vi "Shooter Control and protect.vi"(5 "Shoot":bool, 7 "Reset":bool, 8 "Auto Reset Delay (ms)":dbl, 9 "Target RPM":dbl, 10 "%VBus":dbl, 11 "Talon Status":T1) -> (1 "DISABLED":bool, 2 "Output":dbl, 3 "Control Mode":T2)   [LabVIEW 2016]
doc: "When the shoot terminal recives true the shooter shifts to speed mode and goes to the target speed. When the shoot terminal goes false the shooter stays on for Delay miliseconds. This prevents balls from entering the shooter while it's speed is too low.\n\nWhen the shoot terminal is false the shooter is in manual percent VBus mode.\n\nIf the shooter has stalled it will be disabled. When disabled the shooter will not move and can be re-enabled by sending true to the reset terminal.\n\nThe shooter can also be enabled by using the auto reset. When the Auto reset terminal is set to zero it will not auto reset. When the reset terminal is positive it will wait for The specified delay then set the reset terminal to true."
uses:
  <vilib>/Rock Robotics/WPI/ThirdParty/CanMotor/TalonSRX/WPI_CANTalonSRX_APIControlMode.ctl
  <vilib>/Rock Robotics/WPI/ThirdParty/CanMotor/TalonSRX/WPI_CANTalonSRX_GlobalStatus.ctl
  <vilib>/Rock Robotics/Network Tables/NT Read Boolean.vi
  Delay Polymorphic/Delay Boolean.vi
panel:
  in  "Delay (ms)":i32
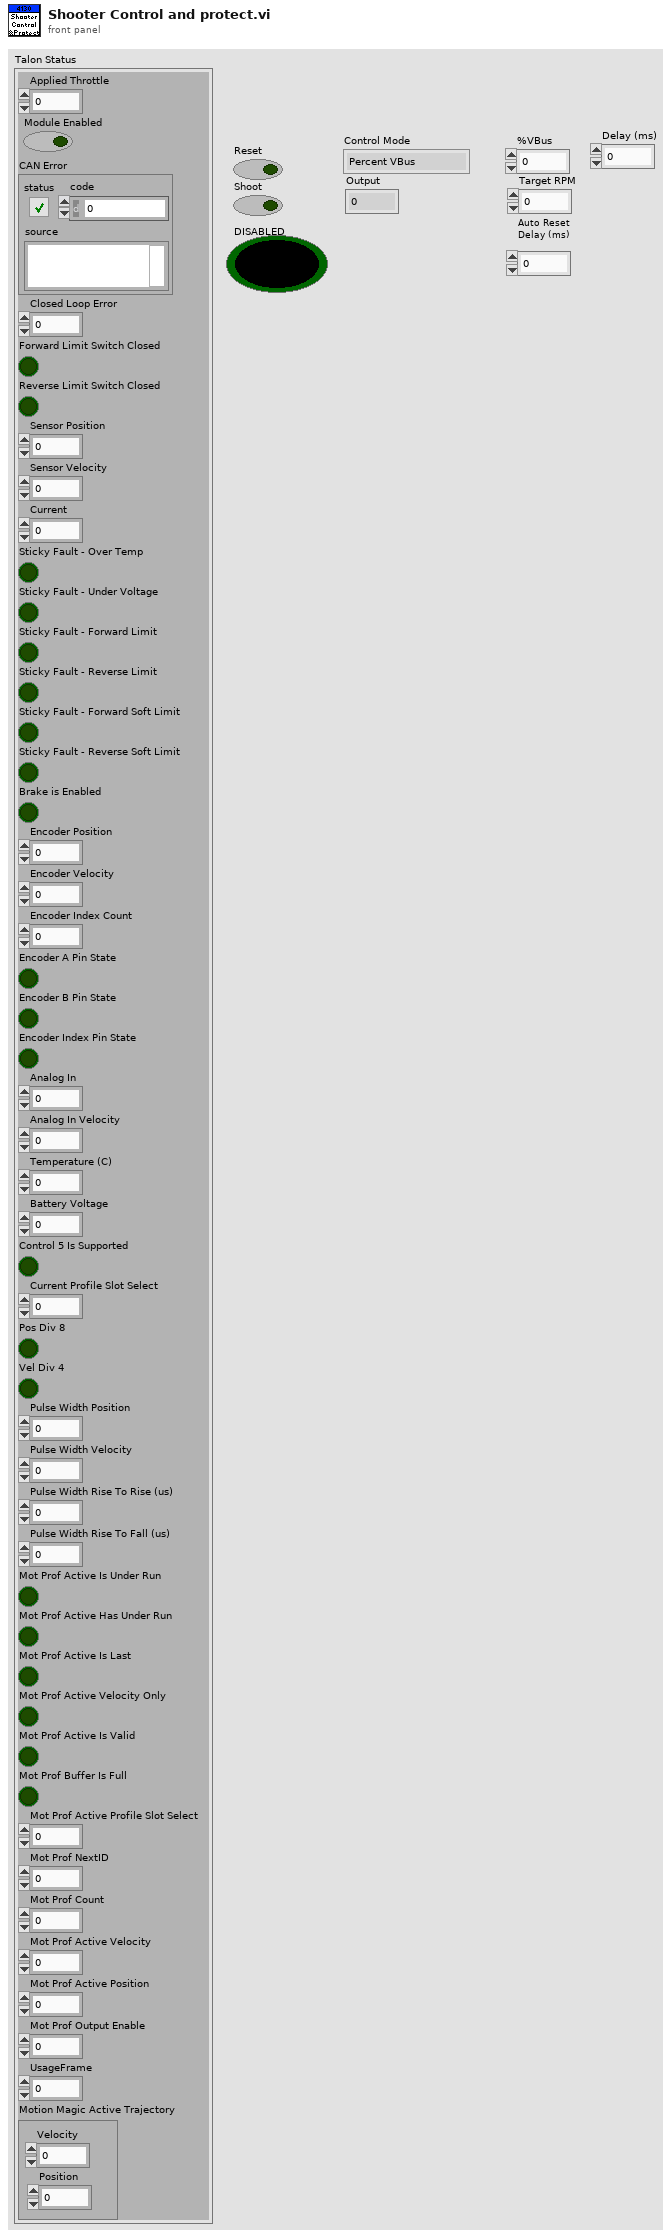
[diagram p1: front panel]
types:
  T1 = typedef "WPI_CANTalonSRX_GlobalStatus.ctl" = cluster{"Applied Throttle":dbl, "Module Enabled":bool, "CAN Error":errorcluster, "Closed Loop Error":dbl, "Forward Limit Switch Closed":bool, "Reverse Limit Switch Closed":bool, "Sensor Position":dbl, "Sensor Velocity":dbl, "Current":dbl, "Sticky Fault - Over Temp":bool, "Sticky Fault - Under Voltage":bool, "Sticky Fault - Forward Limit":bool, "Sticky Fault - Reverse Limit":bool, "Sticky Fault - Forward Soft Limit":bool, "Sticky Fault - Reverse Soft Limit":bool, "Brake is Enabled":bool, "Encoder Position":dbl, "Encoder Velocity":dbl, "Encoder Index Count":dbl, "Encoder A Pin State":bool, "Encoder B Pin State":bool, "Encoder Index Pin State":bool, "Analog In":dbl, "Analog In Velocity":dbl, "Temperature (C)":dbl, "Battery Voltage":dbl, "Control 5 Is Supported":bool, "Current Profile Slot Select":dbl, "Pos Div 8":bool, "Vel Div 4":bool, "Pulse Width Position":i32, "Pulse Width Velocity":i32, "Pulse Width Rise To Rise (us)":i32, "Pulse Width Rise To Fall (us)":i32, "Mot Prof Active Is Under Run":bool, "Mot Prof Active Has Under Run":bool, "Mot Prof Active Is Last":bool, "Mot Prof Active Velocity Only":bool, "Mot Prof Active Is Valid":bool, "Mot Prof Buffer Is Full":bool, "Mot Prof Active Profile Slot Select":i32, "Mot Prof NextID":i32, "Mot Prof Count":i32, "Mot Prof Active Velocity":dbl, "Mot Prof Active Position":dbl, "Mot Prof Output Enable":i32, "UsageFrame":u32, "Motion Magic Active Trajectory":cluster{"Velocity":dbl, "Position":dbl}}
  T2 = typedef "WPI_CANTalonSRX_APIControlMode.ctl" = enum8{"Percent VBus", "Speed", "Position", "Slave", "Unchanged / Invalid", "Voltage Compensation", "Current", "Motion Profile", "Motion Magic"}
  T3 = enum16{"Rising", "Falling", "Neither", "Instant"}
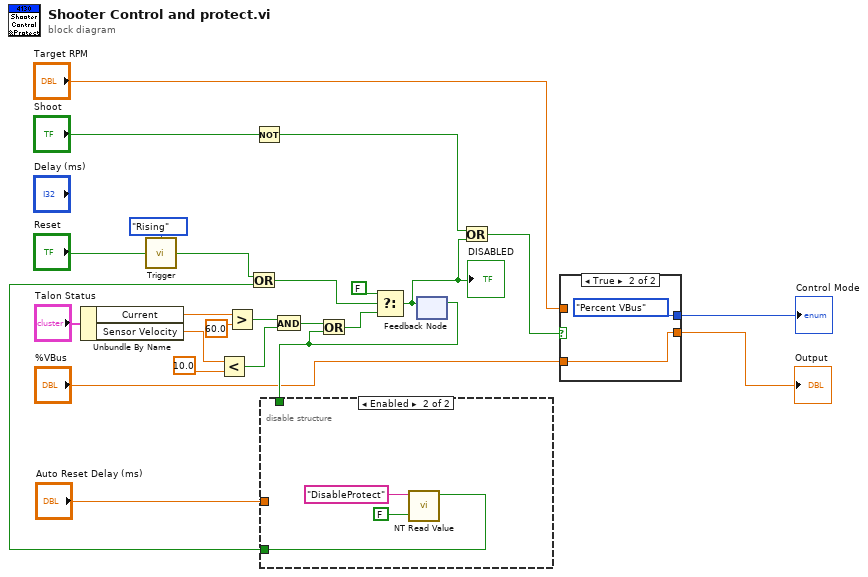
[diagram p0: block diagram]
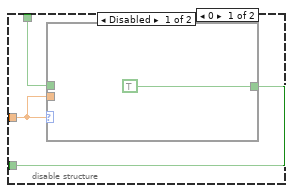
[diagram p2: hidden frame]
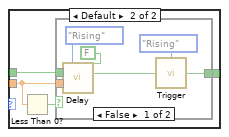
[diagram p3: hidden frame]
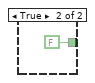
[diagram p4: hidden frame]
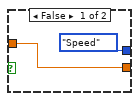
[diagram p5: hidden frame]
diagram:
  n1 = Unbundle By Name("Talon Status") -> ("Current"=w19:dbl, "Sensor Velocity"=w17:dbl)
  n2 = call "Trigger.vi"("Enum"=enum16{"Falling", "Rising", "Both"}."Rising", "Button"="Reset") -> ("Trigger"=w10:bool)  [unwired: 13 in]
  n3 = Less?(x=w17, y=10.0) -> (x < y?=w24:bool)
  n4 = Greater?(x=w19, y=60.0) -> (0:w25:bool)
  n5 = Not(x="Shoot") -> (.not. x?=w2:bool)
  n6 = And(x=w25, y=w24) -> (x .and. y?=w23:bool)
  n7 = feedback #1() -> (w11:bool)  [unwired: 1 in]
  n8 = disable-structure shown="Enabled" {
    disable-tunnel: "Auto Reset Delay (ms)" -> [w28 _]
    disable-tunnel: w11 -> [w27 _]
    disable-tunnel: [w26 w42] -> w9
    frame Disabled {
      n9 = case shown="0" w28 {
        tunnel: w28 -> [_ w31]
        tunnel: w27 -> [_ w33]
        tunnel: [TRUE ("Output") w32] -> w26
        frame 0 {
        }
        frame Default {
          n10 = Less Than 0?(x=w31) -> (x < 0?=w30:bool)
          n11 = case shown="False" w30 {
            tunnel: w33 -> [w40 _]
            tunnel: w31 -> [w39 _]
            tunnel: [w38 FALSE ("Trigger")] -> w32
            frame False {
              n12 = call-poly "Delay.vi"("Mode"=T3."Rising" ("Enum"), "Invert"=FALSE, "input"=w40, "Delay"=w39) -> ("Output"=w34:bool)  [unwired: 9 in, 2 out]
              n13 = call "Trigger.vi"("Enum"=enum16{"Falling", "Rising", "Both"}."Rising", "Button"=w34) -> ("Trigger"=w38:bool)  [unwired: 13 in]
            }
            frame True {
            }
          }
        }
      }
    }
    frame Enabled {
      n14 = call-poly <vilib>:"NT Read Value.vi"("Default Value"=FALSE, "Name"="DisableProtect") -> ("Boolean"=w42:bool)  [unwired: 8 in, 1 out]
    }
  }
  n15 = Or(x=w10, y=w9) -> (x .or. y?=w8:bool)
  n16 = Or(x=w23, y=w11) -> (x .or. y?=w21:bool)
  n17 = Select(t=FALSE, s=w8, f=w21) -> (s? t:f=w4:bool)
  "DISABLED" <- w4
  n18 = feedback-in #1(w4) -> ()
  n19 = Or(x=w2, y=w4) -> (x .or. y?=w15:bool)
  n20 = case shown="True" w15 {
    tunnel: "Target RPM" -> [w45 _]
    tunnel: [WPI_CANTalonSRX_APIControlMode."Speed" ("Control Mode") WPI_CANTalonSRX_APIControlMode."Percent VBus" ("Control Mode")] -> w5
    tunnel: [w45 w47] -> w6
    tunnel: "%VBus" -> [_ w47]
    frame False {
    }
    frame True {
    }
  }
  "Control Mode" <- w5
  "Output" <- w6
